vi "Read Cursor Allow Drag.vi"(8 "error in (no error)":errorcluster, 11 "2D Plot.lvclass in":refnum<class "2D Plot.lvclass">) -> (0 "error out":errorcluster, 2 "Allow Drag":bool, 3 "2D Plot.lvclass out":refnum<class "2D Plot.lvclass">)   [LabVIEW 2020, in "2D Plot.lvclass"]
uses:
  <vilib>/Math Plots/2D Math Plots/2D Plot/2D Plot/2D Plot.lvclass
  <vilib>/Math Plots/2D Math Plots/2D Plot/2D Plot/2D Plot.lvclass/2D Plot.ctl
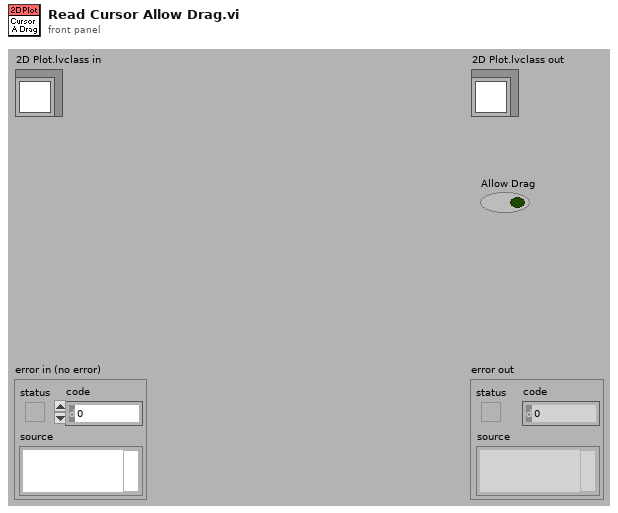
[diagram p1: front panel]
types:
  T1 = typedef "LVCursorListTypeDef.ctl" = cluster{"Name":string, "Color":u32, "Style":u8, "Point Style":u8, "Name Visible":bool, "Allow Drag":bool, "Cursor Mode":u32, "Plot":i32, "Index":i32, "Position":cluster{"X":dbl, "Y":dbl}, "X Scale":u32, "Y Scale":u32, "Watch Plots":i32[], "Watch All Plots":bool, "Plot Area":i32, "Label Offset":cluster{"X":dbl, "Y":dbl}}[]
  T2 = cluster{"Name":string, "Color":u32, "Style":u8, "Point Style":u8, "Name Visible":bool, "Allow Drag":bool, "Cursor Mode":u32, "Plot":i32, "Index":i32, "Position":cluster{"X":dbl, "Y":dbl}, "X Scale":u32, "Y Scale":u32, "Watch Plots":i32[], "Watch All Plots":bool, "Plot Area":i32, "Label Offset":cluster{"X":dbl, "Y":dbl}}
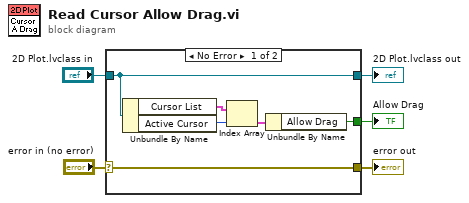
[diagram p0: block diagram]
diagram:
  n1 = case shown="No Error" "error in (no error)" {
    selector: "error in (no error)" -> [w11 w12]
    tunnel: [w11 w12] -> w4
    tunnel: [w7 w13] -> w2
    tunnel: "2D Plot.lvclass in" -> [w7 w13]
    tunnel: [w6 _] -> w1
    frame No Error {
      n2 = Unbundle By Name(w7) -> ("Cursor List"=w10:T1, "Active Cursor"=w8:i32)
      n3 = Index Array(array=w10, index=w8) -> (element=w9:T2)
      n4 = Unbundle By Name(w9) -> ("Allow Drag"=w6:bool)
    }
    frame Error {
    }
  }
  "error out" <- w4
  "2D Plot.lvclass out" <- w2
  "Allow Drag" <- w1
